vi "midi-track.get.vi"(8 "error in (no error)":errorcluster, 10 "Track Number":i32, 11 "midi-file-events in":refnum<class "midi-file-events.lvclass">) -> (0 "error out":errorcluster, 2 "file events":refnum<class "midi-file-event.lvclass">[](array[class]), 3 "midi-file-events out":refnum<class "midi-file-events.lvclass">)   [LabVIEW 2020, in "midi-file-events.lvclass"]
uses:
  midi-file-events.lvclass
  midi-file-event/midi-file-event.lvclass
  midi-file-events.lvclass/midi-file-events.ctl
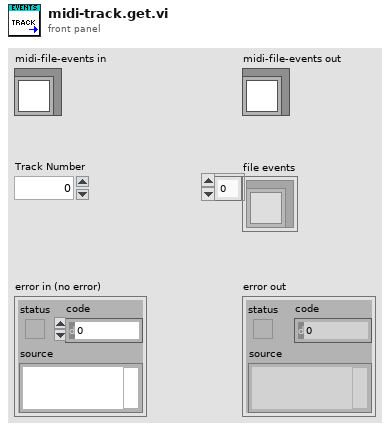
[diagram p1: front panel]
types:
  T1 = map{i32, refnum<class "midi-file-event.lvclass">[]}
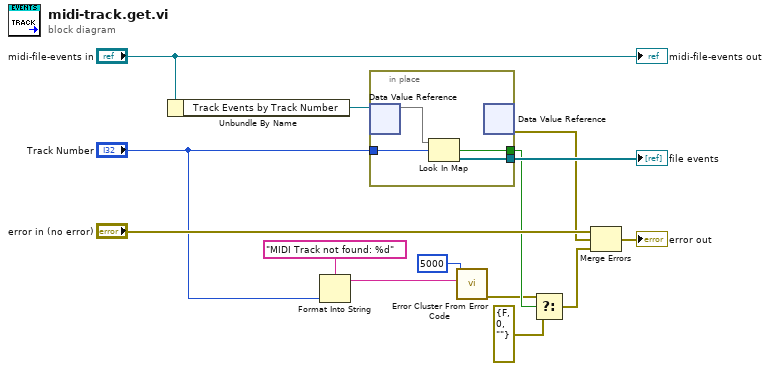
[diagram p0: block diagram]
diagram:
  n1 = Unbundle By Name("midi-file-events in") -> ("Track Events by Track Number"=w14:refnum<data-value>)
  n2 = Format Into String(format string="MIDI Track not found: %d" ("error message (\"\")"), "Track Number") -> (resulting string=w3:string)  [unwired: 2 in, 1 out]
  n3 = in-place {
    in-place-border: "Track Number" -> [w17]
    in-place-border: [w16] -> w13
    in-place-border: [w15] -> w8
    n4 = in-place-dvr #1(w14) -> (w18:T1)  [unwired: 1 out]
    n5 = Look In Map(map=w18, key=w17) -> (key not found?=w15:bool, value=w16:refnum<class "midi-file-event.lvclass">[])  [unwired: 1 in]
    n6 = in-place-dvr #1() -> (w10:errorcluster)  [unwired: 1 in, 1 out]
  }
  "file events" <- w13
  n7 = call <vilib>:"Error Cluster From Error Code.vi"("error message (\"\")"=w3, "error code (0)"=5000) -> ("error out"=w2:errorcluster)  [unwired: 7 in]
  n8 = Select(t=w2, s=w8, f=errorcluster {"status"=FALSE, "code"=0, "source"=""}) -> (s? t:f=w7:errorcluster)
  n9 = Merge Errors("error in (no error)", w10, w7) -> (→"error out":errorcluster)
  "midi-file-events out" <- "midi-file-events in"
